vi "LJUD UE9RAW CommDebug.vi"(7 "Comm Settings":T1={"Open LabJack "=TRUE, "Use USB"=TRUE, "IP Address"="192.168.1.209", "PortA"=52360, "PortB"=0}, 8 "error in (no error)":errorcluster, 11 "Handle In":i32) -> (0 "error out":errorcluster, 3 "Handle Out":i32)   [LabVIEW 2021]
panel:
  out "Heap Space":u16
  out "Write Array":u8[](array[numeric]) format="%.0x"
  out "Read Array":u8[](array[numeric]) format="%.0x"
  # "15"
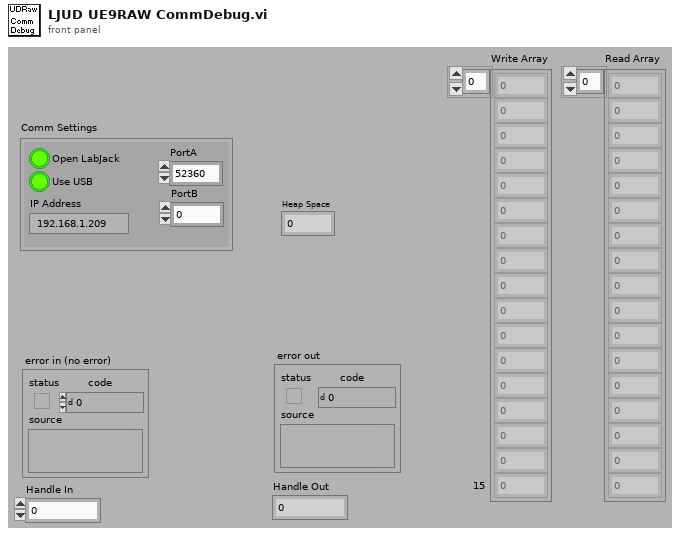
[diagram p1: front panel]
types:
  T1 = cluster{"Open LabJack ":bool, "Use USB":bool, "IP Address":string, "PortA":u16, "PortB":u16}
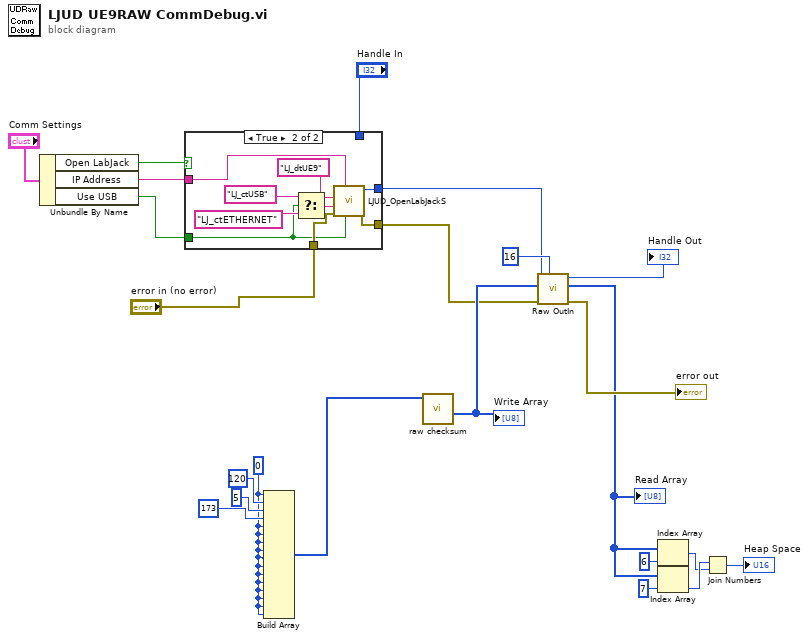
[diagram p0: block diagram]
diagram:
  w3 = u8 0 ("Input Element")
  n1 = Unbundle By Name("Comm Settings") -> ("Open LabJack"=w4:bool, "IP Address"=w5:string, "Use USB"=w6:bool)
  n2 = case shown="True" w4 {
    tunnel: w5 -> [_ w28]
    tunnel: "error in (no error)" -> [w25 w32]
    tunnel: [w25 w31] -> w8
    tunnel: [w24 w29] -> w9
    tunnel: w6 -> [_ w30]
    tunnel: "Handle In" -> [w24 _]
    frame False {
    }
    frame True {
      n3 = Select(t="LJ_ctUSB" ("ConnectionType"), s=w30, f="LJ_ctETHERNET" ("ConnectionType")) -> (s? t:f=w26:string)
      n4 = call "LJUD_OpenLabJackS.vi"("FirstFound"=w30, "Address"=w28, "error in"=w32, "ConnectionType"=w26, "DeviceType"="LJ_dtUE9") -> ("error out"=w31:errorcluster, "Handle"=w29:i32)  [unwired: 4 in, 1 out]
    }
  }
  n5 = Build Array(w3, u8 120 ("Input Element"), u8 5 ("Input Element"), u8 173 ("Input Element"), w3, w3, w3, w3, w3, w3, w3, w3, w3, w3, w3, w3) -> (w16:u8[])
  n6 = call "raw checksum.vi"("Array"=w16) -> ("Array Output"=w15:u8[])  [unwired: 3 in, 7 out]
  "Write Array" <- w15
  n7 = call "Raw OutIn.vi"("# of bytes to read in"=16 ("# of bytes to read"), "error in"=w8, "Raw Out"=w15, "Handle In"=w9) -> ("error out"=→"error out":errorcluster, "Raw In"=w2:u8[], "Handle Out"=→"Handle Out":i32)  [unwired: 4 in, 1 out]
  "Read Array" <- w2
  n8 = Index Array(array=w2, index=6 ("Index")) -> (element=w17:u8)
  n9 = Index Array(array=w2, index=7 ("Index")) -> (element=w18:u8)
  n10 = Join Numbers(hi=w18, lo=w17) -> ((hi.lo)=→"Heap Space":u16)
